vi "Unsubscribe (Array).vi"(6 "timeout (1000ms)":i32=1000, 8 "error in (no error)":errorcluster, 10 "Topics":string[](array[string]), 11 "Client in":refnum<class "Client.lvclass">) -> (0 "error out":errorcluster, 3 "Client out":refnum<class "Client.lvclass">)   [LabVIEW 2013, in "MQTT Client.lvlib" / "Client.lvclass"]
uses:
  Client.lvclass
  <vilib>/LabVIEW Open Source Project/MQTT Connection/MQTT_Base/Base Class/MQTT_Base.lvclass
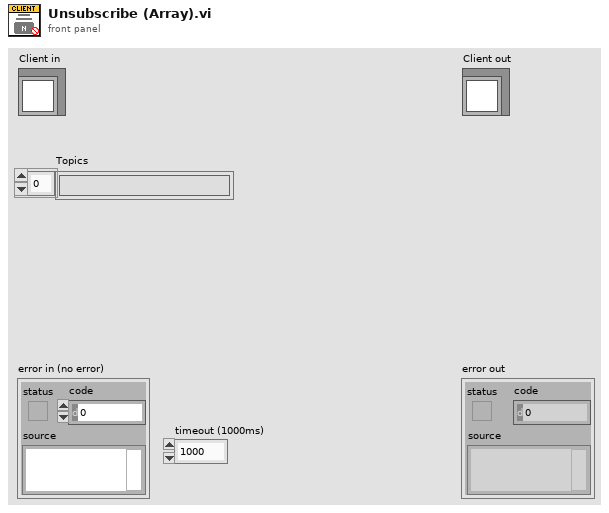
[diagram p1: front panel]
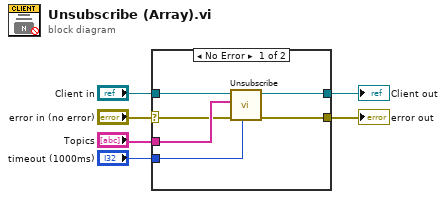
[diagram p0: block diagram]
diagram:
  n1 = case shown="No Error" "error in (no error)" {
    selector: "error in (no error)" -> [w7 w14]
    tunnel: [w10 w14] -> w5
    tunnel: [w11 w13] -> w3
    tunnel: "Client in" -> [w12 w13]
    tunnel: "Topics" -> [w8 _]
    tunnel: "timeout (1000ms)" -> [w9 _]
    frame No Error {
      n2 = call <vilib>:"Unsubscribe.vi"("timeout (1000 ms)"=w9, "error in (no error)"=w7, "Topics"=w8, "MQTT_Base in"=w12) -> ("error out"=w10:errorcluster, "MQTT_Base out"=w11:refnum<class "Client.lvclass">)  [unwired: 5 in, 1 out]
    }
    frame Error {
    }
  }
  "error out" <- w5
  "Client out" <- w3
